vi "Get Sensor Number.vi"(8 "error in (no error)":errorcluster, 11 "Sensor Number Msg in":refnum<class "Sensor Number Msg.lvclass">) -> (0 "error out":errorcluster, 2 "Sensor Number":i32, 3 "Sensor Number Msg out":refnum<class "Sensor Number Msg.lvclass">)   [LabVIEW 2013, in "Main Model.lvlib" / "Sensor Number Msg.lvclass"]
uses:
  Sensor Number Msg.lvclass
  Sensor Number Msg.lvclass/Sensor Number Msg.ctl
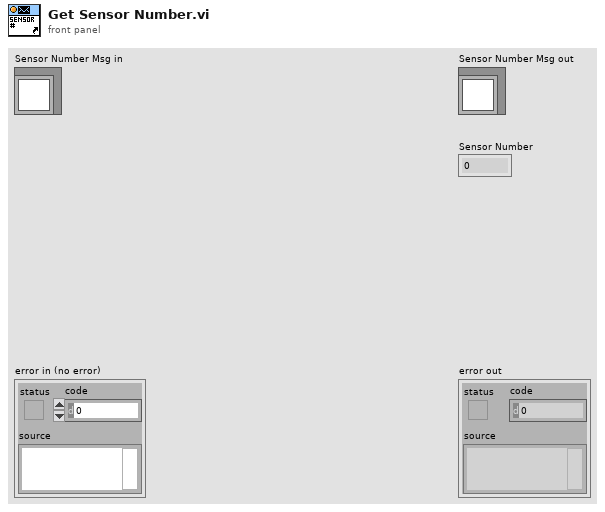
[diagram p1: front panel]
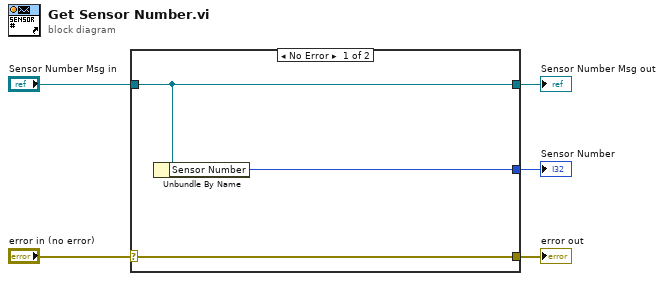
[diagram p0: block diagram]
diagram:
  n1 = case shown="No Error" "error in (no error)" {
    selector: "error in (no error)" -> [w8 w9]
    tunnel: [w8 w9] -> w4
    tunnel: [w7 w10] -> w2
    tunnel: "Sensor Number Msg in" -> [w7 w10]
    tunnel: [w6 _] -> w1
    frame No Error {
      n2 = Unbundle By Name(w7) -> ("Sensor Number"=w6:i32)
    }
    frame Error {
    }
  }
  "error out" <- w4
  "Sensor Number Msg out" <- w2
  "Sensor Number" <- w1
